vi "read-&-parse-visa.vi"(6 "Bytes at Port":u32, 7 "Command":T1, 8 "error in (no error)":errorcluster, 9 "Analog Data in":T3, 10 "Thermocouples in":T2, 11 "VISA Refnum in":refnum<visa-resource-name>) -> (0 "error out":errorcluster, 1 "Analog Data out":T3, 2 "Thermocouples out":T2, 3 "VISA Refnum out":refnum<visa-resource-name>, 4 "status  out":string)   [LabVIEW 2024]
uses:
  controls/depreciated/analog-data-cluster.ctl
  controls/depreciated/thermocouple-data-cluster.ctl
  controls/command-enum.ctl
panel:
  out "read buffer":string
  out "acknowledge char":string
  out "read return":u32
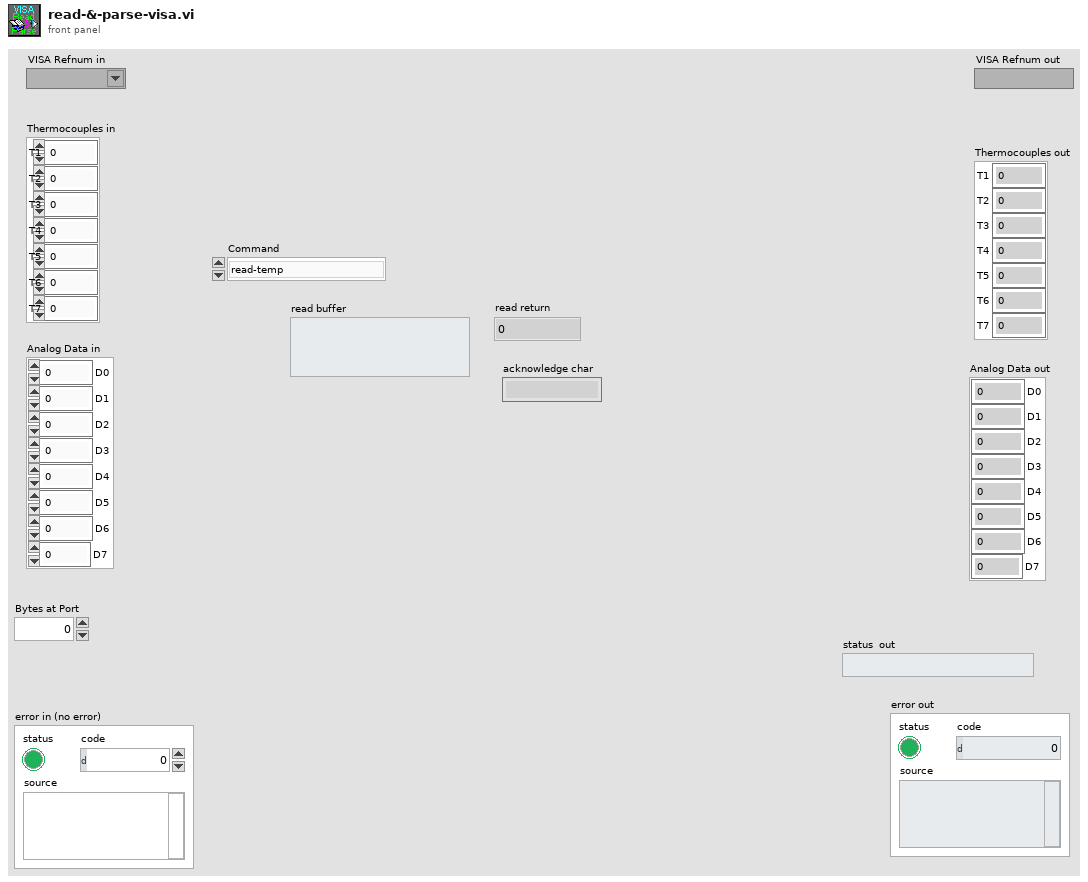
[diagram p1: front panel]
types:
  T1 = typedef "command-enum.ctl" = enum16{"read-temp", "read-AI"}
  T2 = typedef "thermocouple-data-cluster.ctl" = cluster{"T1":dbl, "T2":dbl, "T3":dbl, "T4":dbl, "T5":dbl, "T6":dbl, "T7":dbl}
  T3 = typedef "analog-data-cluster.ctl" = cluster{"D0":dbl, "D1":dbl, "D2":dbl, "D3":dbl, "D4":dbl, "D5":dbl, "D6":dbl, "D7":dbl}
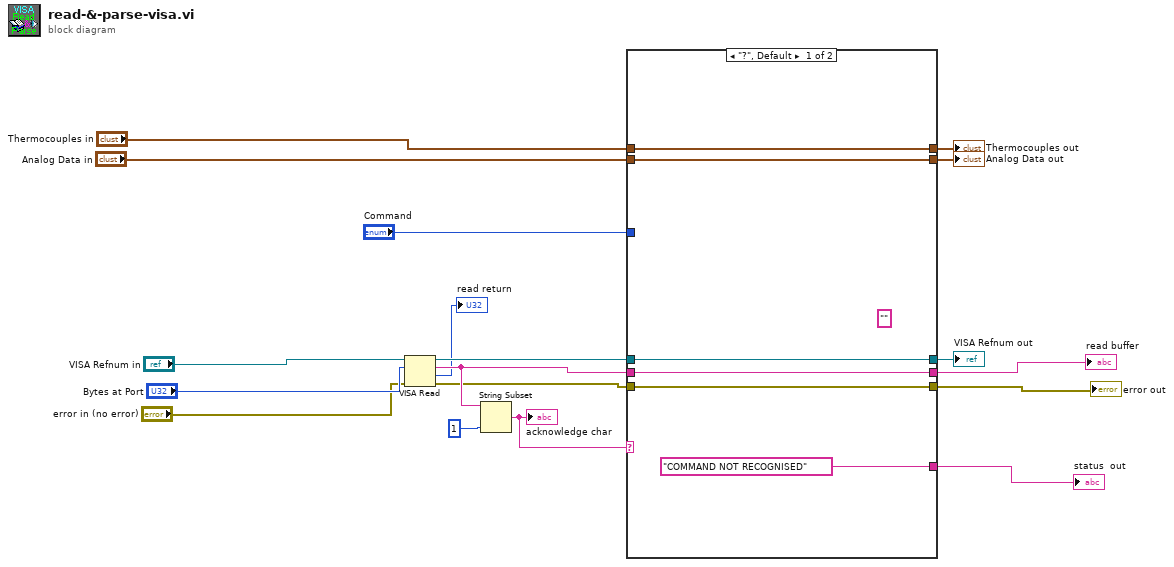
[diagram p0: block diagram]
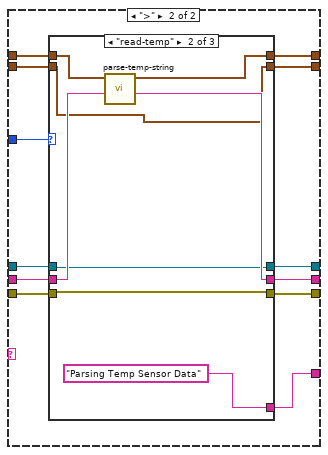
[diagram p2: hidden frame]
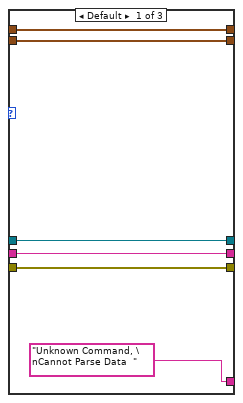
[diagram p3: hidden frame]
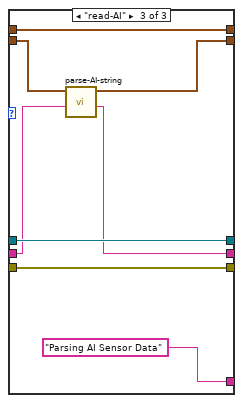
[diagram p4: hidden frame]
diagram:
  n1 = VISA Read(VISA resource name="VISA Refnum in", byte count="Bytes at Port", error in (no error)="error in (no error)") -> (VISA resource name out=w14:refnum<visa-resource-name>, read buffer=w16:string, return count=→"read return":u32, error out=w15:errorcluster)
  n2 = String Subset(string=w16, length (rest)=1 ("length (rest)")) -> (substring=w18:string)  [unwired: 1 in]
  "acknowledge char" <- w18
  n3 = case shown="\"?\", Default" w18 {
    tunnel: "Command" -> [_ w36]
    tunnel: [w21 w35] -> w2
    tunnel: [w22 w34] -> w3
    tunnel: [w20 w33] -> w4
    tunnel: [w24 w32] -> w5
    tunnel: ["COMMAND NOT RECOGNISED" ("status") w31] -> w6
    tunnel: "Thermocouples in" -> [w24 w30]
    tunnel: "Analog Data in" -> [w23 w29]
    tunnel: [w23 w28] -> w9
    tunnel: w14 -> [w22 w27]
    tunnel: w15 -> [w20 w26]
    tunnel: w16 -> [w21 w25]
    frame "?", Default {
      (unwired) "" ("csv")
    }
    frame ">" {
      n4 = case shown="\"read-temp\"" w36 {
        tunnel: w25 -> [w39 w47 w54]
        tunnel: [w39 w46 w53] -> w35
        tunnel: w27 -> [w41 w44 w58]
        tunnel: [w41 w44 w58] -> w34
        tunnel: [w40 w43 w57] -> w33
        tunnel: w26 -> [w40 w43 w57]
        tunnel: ["Unknown Command, \nCannot Parse Data  " ("status") "Parsing Temp Sensor Data" ("status") "Parsing AI Sensor Data" ("status")] -> w31
        tunnel: [w38 w50 w51] -> w32
        tunnel: w30 -> [w38 w48 w51]
        tunnel: w29 -> [w37 w45 w55]
        tunnel: [w37 w45 w52] -> w28
        frame Default {
        }
        frame "read-temp" {
          n5 = call "parse-temp-string.vi"("read buffer in"=w47, "Thermocouples"=w48) -> ("csv"=w46:string, "Thermocouples"=w50:T2)  [unwired: 8 in]
        }
        frame "read-AI" {
          n6 = call "parse-AI-string.vi"("read buffer in"=w54, "Analog Data"=w55) -> ("csv"=w53:string, "Analog Data Out"=w52:T3)  [unwired: 8 in]
        }
      }
    }
  }
  "Analog Data out" <- w9
  "status  out" <- w6
  "Thermocouples out" <- w5
  "VISA Refnum out" <- w3
  "read buffer" <- w2
  "error out" <- w4
